vi "ShouldDisplay.vi"(8 "error in (no error)":errorcluster, 10 "verbosity":T1, 11 "errorSeverity":T1) -> (0 "error out":errorcluster, 3 "dialogType":i32)   [LabVIEW 2026, in "Lumberjack.lvlib"]
doc: "Pure verbosity-gate decision: maps a caught error's severity and the current verbosity setting to the General Error Handler \"type of dialog\" selector, so the display decision is unit-testable apart from any modal (SRS-LMBR-042).\nReturns dialogType 1 (OK message, shown) when the error is at least as severe as the verbosity threshold, i.e. rank(errorSeverity) <= rank(verbosity) via RankCompare; otherwise 0 (no dialog). Verbosity is itself a Severity threshold, so ALL shows every dialog and OFF (the launch default) shows none.\nGoverns display only; logging is independent and unaffected by this result.\nLumberjack.lvlib, public; called by Logger.CatchError (errorSeverity = ERROR, verbosity from GetVerbosity) and the LMBR-T-055 unit test. No state, no I/O; deterministic."
uses:
  Lumberjack.lvlib
  TypeDefs/Severity.ctl
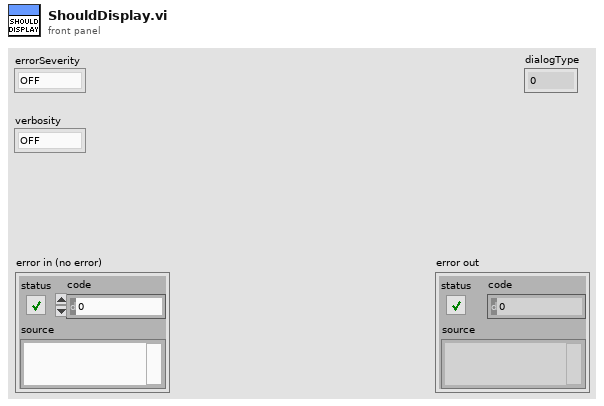
[diagram p1: front panel]
types:
  T1 = typedef "Lumberjack.lvlib/Severity.ctl" = enum16{"OFF", "FATAL", "ERROR", "WARN", "INFO", "DEBUG", "TRACE", "ALL"}
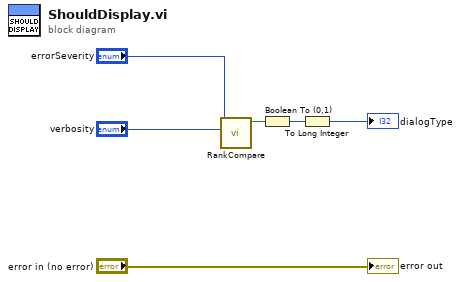
[diagram p0: block diagram]
diagram:
  n1 = call "RankCompare.vi"("Threshold"="verbosity", "Level"="errorSeverity") -> ("Passes"=w3:bool)  [unwired: 8 in, 1 out]
  n2 = Boolean To (0,1)(Boolean=w3) -> (0, 1=w2:i16)
  n3 = To Long Integer(number=w2) -> (32bit integer=→"dialogType":i32)
  "error out" <- "error in (no error)"
